vi "Show Brief Status.vi"() -> ()   [LabVIEW 2018]
uses:
  Type/_Source Type.ctl
  Type/_RT Command.ctl
  Type/_Log Command.ctl
  Configuration/_Global Configuration.vi
panel:
  out "Vac. Pressure:":sgl format="%#.2e"
  out "Source 1 Type:":T1 items=["None", "ESI", "APCI", "APPI", "MicroSpray"]
  out "Source 2 Type:":T1 items=["None", "ESI", "APCI", "APPI", "MicroSpray"]
  out "Heaters Temp:":sgl caption="P1 T" format="%#.2g"
  out "Flange Temp:":sgl caption="P2 T" format="%#.2g"
  out "HSID Temp:":sgl format="%#.2g"
  out "Interlock OK":bool
  out "CurGas OK":bool
  out "Pump OK":bool
  out "Exhaust OK":bool
  out "Read":bool
  out "RT Events":string
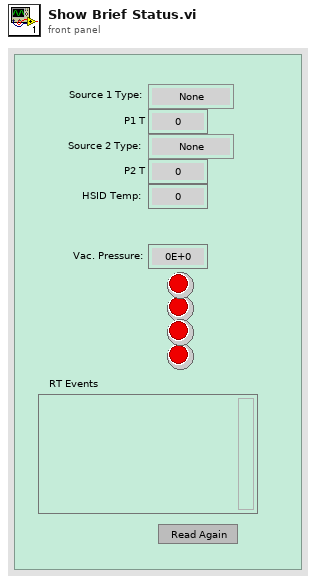
[diagram p1: front panel]
types:
  T1 = typedef "_Source Type.ctl" = i8
  T2 = typedef "_RT Command.ctl" = enum16{"xml Start Run", "xml Start Actual Run", "xml Stop Run", "xml Runtime Update", "xml Get Status", "xml Get Table", "xml Set Table", "xml Get Configuration", "xml System Status", "xml Set LC Input Logic", "xml Get Data", "xml Get Info", "Start", "StartActualRun", "Stop", "Runtime Update", "Get Data", "Get Info", "Get Status", "Get Param", "Get Config", "Get Table", "Read ADC", "Set Oscillator", "Update Config", "Update Table", "Set All Pol", "Set Pol and DC", "Set Max Mass", "Toggle RP", "Toggle EL", "Set PIC", "Initialize Turbo", "Send Turbo Comm", "Close Turbo", "P1", "P2", "P3", "Send Serial", "Set LC Out", "Get LC In", "Read VAC", "Test Table", "Toggle Power", "Get Startup", "Set Startup", "Get ADC Table", "Set ADC Table", "Get Brief Status", "Get Detail Status", "Auxiliary Update", "Set CC Logics", "Set CC Input Logics", "Ignore Error", "invalid"}
  T3 = typedef "_Log Command.ctl" = enum16{"No Command", "Open", "Read", "Write", "Close", "Check Size"}
  T4 = typedef "_RT Instrument 2.ctl" = cluster{"Table":T5[], "Instrument":string[]}
  T5 = typedef "_RT Configuration 2.ctl" = cluster{"Name":string, "Ch#":u8, "Min":dbl, "Max":dbl, "Def+":dbl, "Def-":dbl, "Offset":dbl, "Slope":dbl, "Type":u8, "Description":string, "SettleT":dbl}
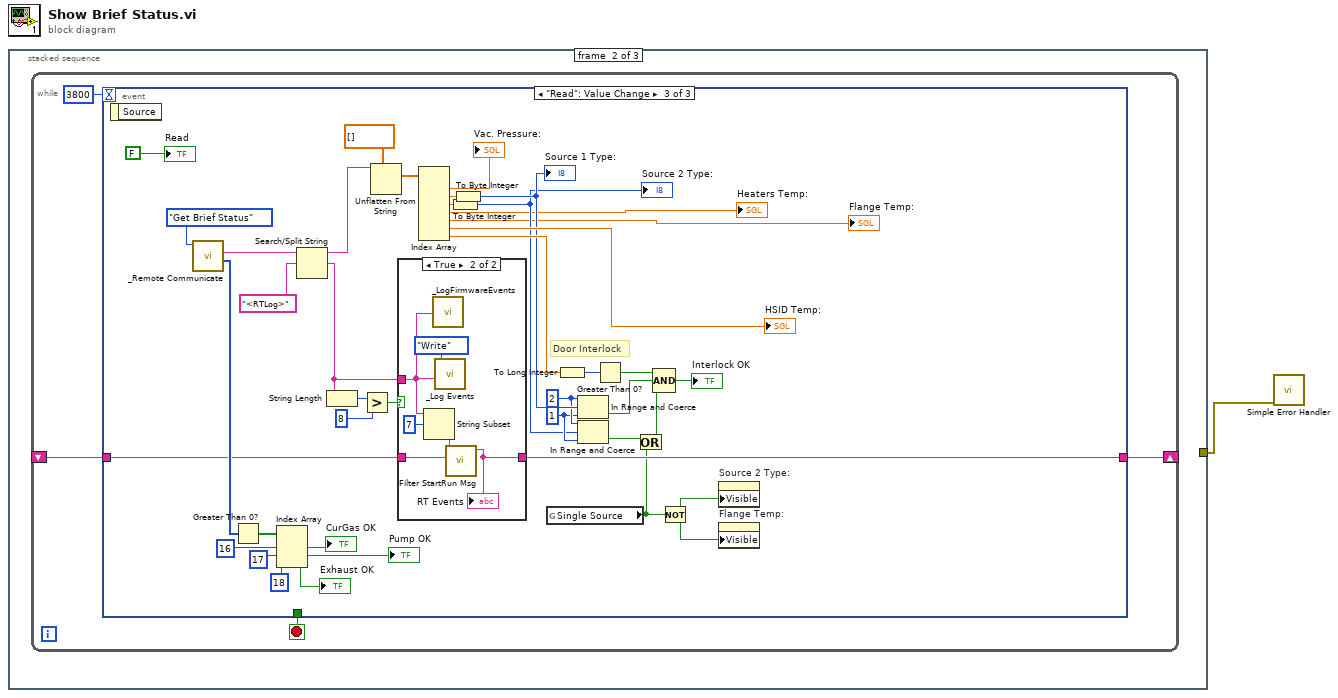
[diagram p0: block diagram]
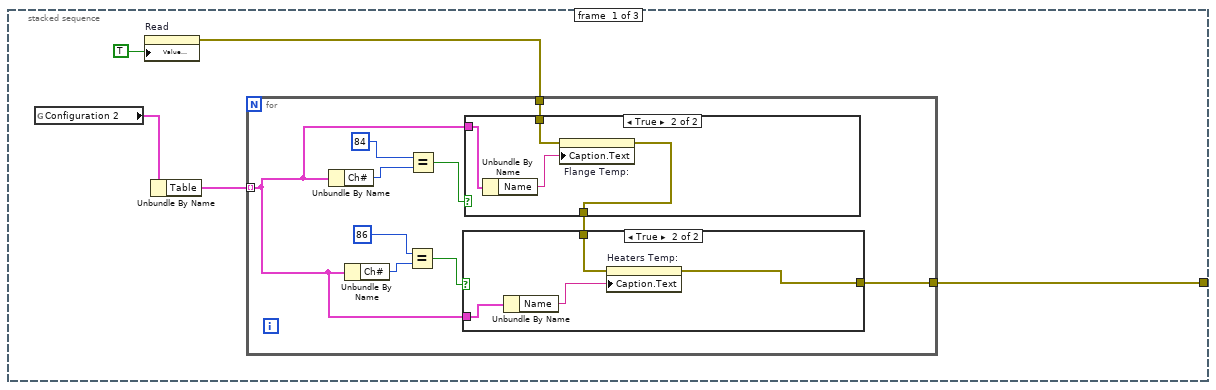
[diagram p2: hidden frame]
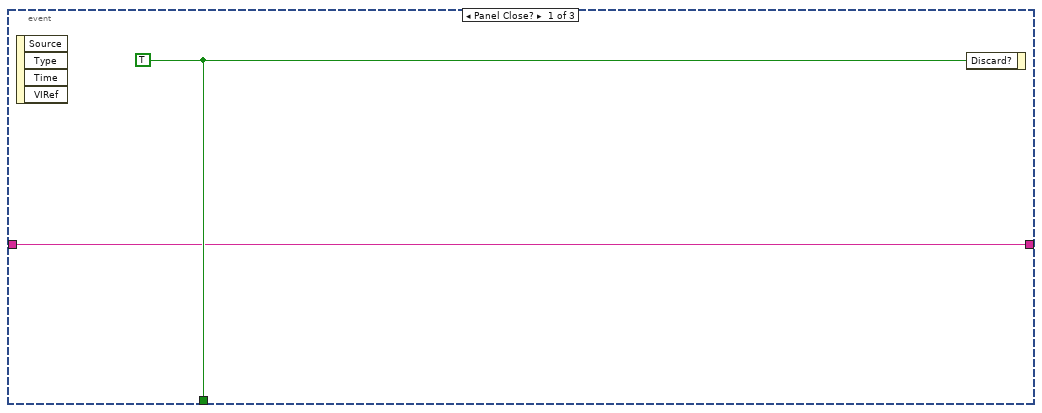
[diagram p5: hidden frame]
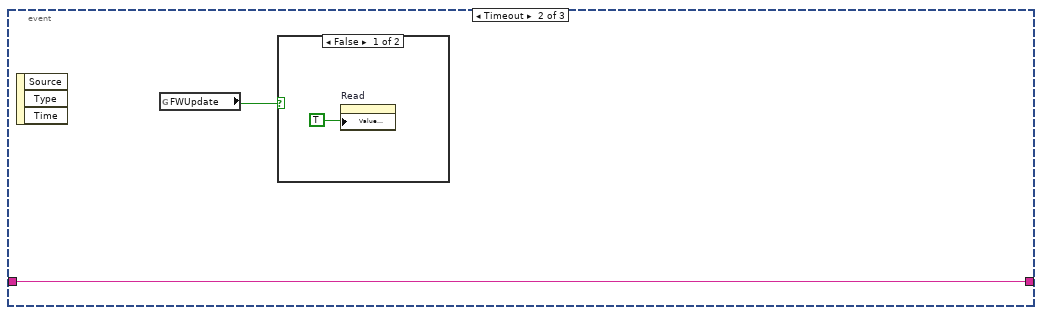
[diagram p6: hidden frame]
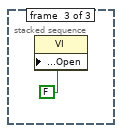
[diagram p9: hidden frame]
diagram:
  n1 = stacked-sequence {
    tunnel: [w2 _ _] -> w1
    frame #0 {
      n2 = global read "_Global Configuration.vi" "Configuration 2"() -> (w5:T4)
      n3 = property on="Read" class="Bool (strict)"("Value (Signaling)"=TRUE) -> (error out=w3:errorcluster)  [unwired: 2 in, 1 out]
      n4 = Unbundle By Name(w5) -> ("Table"=w4:T5[])
      n5 = for {
        tunnel: w4 -> [w7] mode=indexing
        tunnel: w3 -> [w15]
        tunnel: [w14] -> w2
        n6 = Unbundle By Name(w7) -> ("Ch#"=w10:u8)
        n7 = Unbundle By Name(w7) -> ("Ch#"=w11:u8)
        n8 = Equal?(x=u8 86 ("y"), y=w11) -> (x = y?=w12:bool)
        n9 = Equal?(x=u8 84 ("y"), y=w10) -> (x = y?=w13:bool)
        n10 = case shown="True" w13 {
          tunnel: [w22 w23] -> w16
          tunnel: w15 -> [w22 w26]
          tunnel: w7 -> [_ w25]
          frame False {
          }
          frame True {
            n11 = Unbundle By Name(w25) -> ("Name"=w24:string)
            n12 = property on="Flange Temp:" class="DigNum (strict)"(error in=w26, "Caption.Text"=w24) -> (error out=w23:errorcluster)  [unwired: 1 in, 1 out]
          }
        }
        n13 = case shown="True" w12 {
          tunnel: w16 -> [w17 w21]
          tunnel: [w17 w18] -> w14
          tunnel: w7 -> [_ w20]
          frame False {
          }
          frame True {
            n14 = Unbundle By Name(w20) -> ("Name"=w19:string)
            n15 = property on="Heaters Temp:" class="DigNum (strict)"(error in=w21, "Caption.Text"=w19) -> (error out=w18:errorcluster)  [unwired: 1 in, 1 out]
          }
        }
      }
    }
    frame #1 {
      n16 = while {
        shift-right: [w27] -> _
        shift-left: _ -> [w28]
        stop <- w30 stop-if-true
        n17 = event shown="[2] \"Read\": Value Change" {
          selector: _ -> [_ _ _]
          dyn-events: _ -> [_ _ _]
          timeout: 3800 -> [_ _ _]
          tunnel: [w32 _ _] -> w30
          tunnel: w28 -> [w31 w34 w50]
          tunnel: [w31 w34 w49] -> w27
          event Panel Close? {
            w32 = TRUE ("Discard?")
            n18 = event-data() -> ()  [unwired: 5 out]
            n19 = event-data("Discard?"=w32) -> ()  [unwired: 1 in, 1 out]
          }
          event Timeout {
            n20 = event-data() -> ()  [unwired: 4 out]
            n21 = global read "_Global Configuration.vi" "FWUpdate"() -> (w33:bool)
            n22 = case shown="False" w33 {
              frame False {
                n23 = property on="Read" class="Bool (strict)"("Value (Signaling)"=TRUE) -> ()  [unwired: 2 in, 2 out]
              }
              frame True {
              }
            }
          }
          event "Read": Value Change {
            w62 = i8 1 ("lower limit")
            w63 = i8 2 ("upper limit")
            # "Door Interlock"
            n24 = event-data() -> ()  [unwired: 2 out]
            n25 = call "_Remote Communicate.vi"("Command"=_RT_Command."Get Brief Status") -> ("Data Array"=w73:i32[], "Info"=w57:string)  [unwired: 5 in, 2 out]
            n26 = Greater Than 0?(x=w73) -> (x > 0?=w67:bool[])
            n27 = Index Array(array=w67, index #1=16 ("index"), index #2=17 ("index"), index #3=18 ("index")) -> (element #1=→"CurGas OK":bool, element #2=→"Pump OK":bool, element #3=→"Exhaust OK":bool)
            n28 = Search/Split String(string=w57, search string/char (-)="<RTLog>") -> (substring before match=w55:string, match + rest of string=w52:string)  [unwired: 2 out]
            n29 = String Length(string=w52) -> (length=w54:i32)
            n30 = Greater?(x=w54, y=8) -> (0:w51:bool)
            n31 = Unflatten From String(type=sgl[] [], binary string=w55) -> (value=w72:sgl[])  [unwired: 1 in, 4 out]
            n32 = case shown="True" w51 {
              tunnel: w52 -> [_ w80]
              tunnel: w50 -> [w76 w79]
              tunnel: [w76 w78] -> w49
              frame False {
              }
              frame True {
                n33 = String Subset(string=w80, offset (0)=7) -> (substring=w77:string)  [unwired: 1 out]
                n34 = call "_LogFirmwareEvents.vi"("Event"=w80) -> ()
                n35 = call "_Log Events.vi"("Event"=w80, "Log Command"=_Log_Command."Write" ("File Command")) -> ()  [unwired: 6 in, 2 out]
                n36 = call "Filter StartRun Msg.vi"("Current List"=w79, "New RT Events"=w77) -> ("New List"=w78:string)  [unwired: 9 in]
                "RT Events" <- w78
              }
            }
            n37 = Index Array(array=w72) -> (element #1=→"Vac. Pressure:":sgl, element #2=w65:sgl, element #3=w71:sgl, element #4=→"Heaters Temp:":sgl, element #5=→"Flange Temp:":sgl, element #6=→"HSID Temp:":sgl, element #7=w68:sgl)  [unwired: 7 in]
            n38 = To Byte Integer(number=w71) -> (8bit integer=w61:i8)
            "Source 2 Type:" <- w61
            n39 = To Byte Integer(number=w65) -> (8bit integer=w64:i8)
            "Source 1 Type:" <- w64
            n40 = global read "_Global Configuration.vi" "Single Source"() -> (w46:bool)
            n41 = To Long Integer(number=w68) -> (32bit integer=w69:i32)
            n42 = In Range and Coerce(upper limit=w63, x=w64, lower limit=w62) -> (In Range?=w59:bool)  [unwired: 1 out]
            n43 = In Range and Coerce(upper limit=w63, x=w61, lower limit=w62) -> (In Range?=w47:bool)  [unwired: 1 out]
            n44 = Greater Than 0?(x=w69) -> (x > 0?=w60:bool)
            n45 = Or(x=w47, y=w46) -> (x .or. y?=w45:bool)
            n46 = Compound Arithmetic op=AND(w60, w59, w45) -> (→"Interlock OK":bool)
            n47 = Not(x=w46) -> (.not. x?=w48:bool)
            n48 = property on="Source 2 Type:" class="Ring (strict)"("Visible"=w48) -> ()  [unwired: 2 in, 2 out]
            n49 = property on="Flange Temp:" class="DigNum (strict)"("Visible"=w48) -> ()  [unwired: 2 in, 2 out]
            "Read" <- FALSE ("Undo")
          }
        }
      }
    }
    frame #2 {
      n50 = property class="VI"("Front Panel.Open"=FALSE ("Front Panel Window:Open")) -> ()  [unwired: 2 in, 2 out]
    }
  }
  n51 = call <vilib>:"Simple Error Handler.vi"("error in (no error)"=w1) -> ()  [unwired: 4 in, 5 out]
